vi "Format Address.vi"(8 "error in (no error)":errorcluster, 11 "Address":string) -> (0 "error out":errorcluster, 3 "Formatted Address":string)   [LabVIEW 2025, in "Power Supply.lvlib" / "Lambda Gen LAN.lvclass"]
uses:
  Lambda Gen LAN.lvclass
  Lambda Gen LAN.lvclass/Lambda Gen LAN.ctl
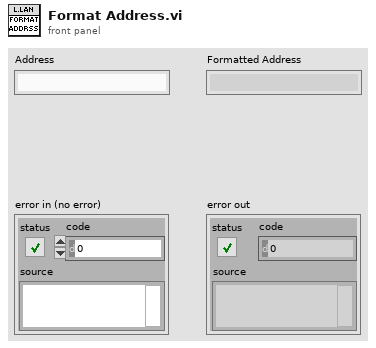
[diagram p1: front panel]
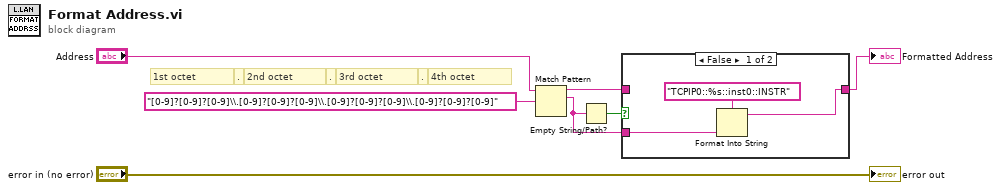
[diagram p0: block diagram]
diagram:
  # "."
  # "."
  # "."
  # "4th octet"
  # "3rd octet"
  # "2nd octet"
  # "1st octet"
  n1 = Match Pattern(string="Address", regular expression="[0-9]?[0-9]?[0-9]\\.[0-9]?[0-9]?[0-9]\\.[0-9]?[0-9]?[0-9]\\.[0-9]?[0-9]?[0-9]" ("format string")) -> (before substring=w2:string, match substring=w4:string)  [unwired: 1 in, 2 out]
  n2 = Empty String/Path?(string/path=w4) -> (empty?=w5:bool)
  n3 = case shown="False" w5 {
    tunnel: w4 -> [w9 _]
    tunnel: [w8 w11] -> w3
    tunnel: w2 -> [_ w11]
    frame False {
      n4 = Format Into String(format string="TCPIP0::%s::inst0::INSTR", w9) -> (resulting string=w8:string)  [unwired: 2 in, 1 out]
    }
    frame True {
    }
  }
  "Formatted Address" <- w3
  "error out" <- "error in (no error)"
